vi "DIO - Set Digital Output.vi"(8 "error in":errorcluster, 10 "Channel Number":i32, 11 "TCP Network Connection in":refnum<k5>) -> (0 "error out":errorcluster, 3 "TCP Network Connection out":refnum<k5>)   [LabVIEW 2020]
doc: "Set the state of a digital output. Before setting the state, the channel direction must be set to output."
panel:
  in  "State":bool
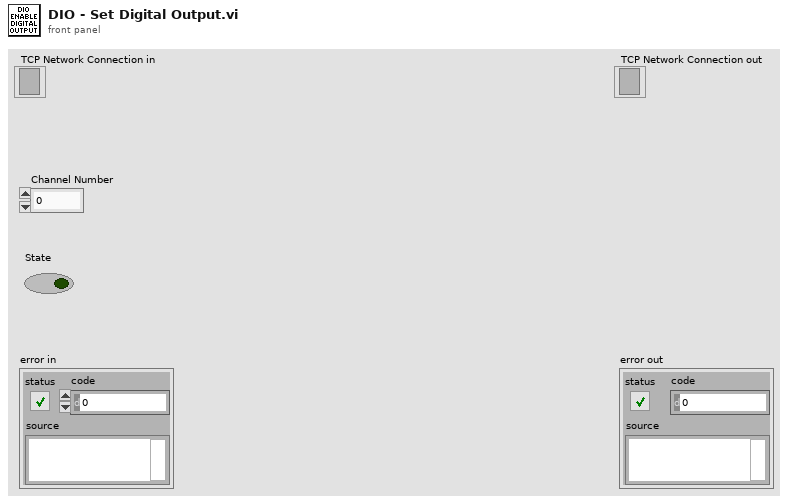
[diagram p1: front panel]
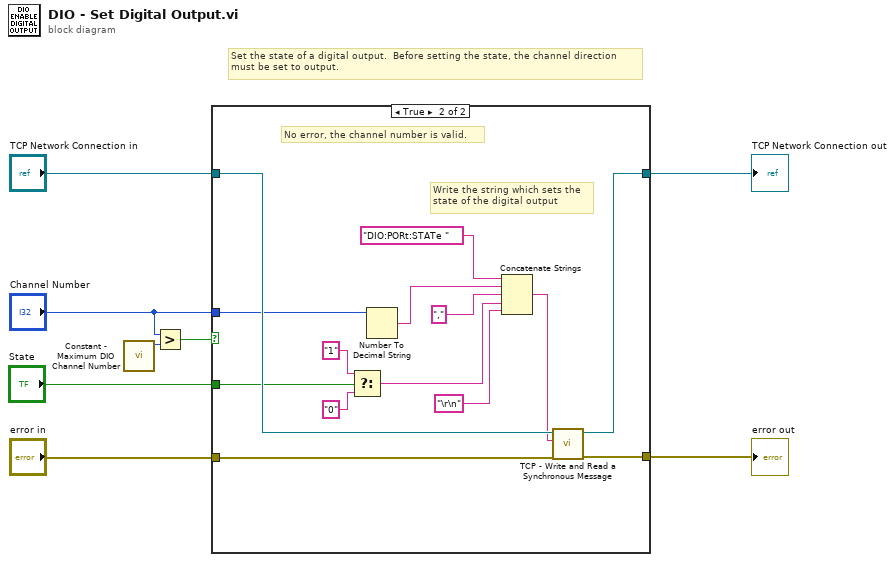
[diagram p0: block diagram]
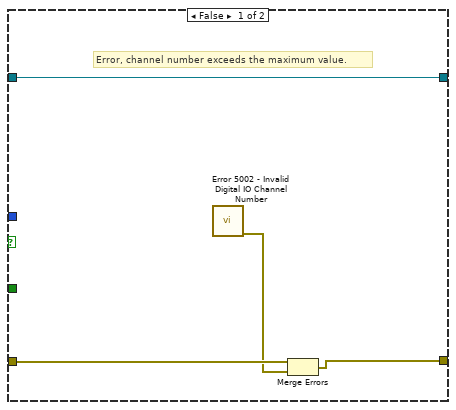
[diagram p2: hidden frame]
diagram:
  # "Set the state of a digital output.  Before setting the state, the channel direction\nmust be set to output."
  n1 = call "Constant - Maximum DIO Channel Number.vi"() -> ("Maximum Channel"=w2:i32)  [unwired: 11 in]
  n2 = Greater?(x="Channel Number", y=w2) -> (0:w1:bool)
  n3 = case shown="True" w1 {
    tunnel: "error in" -> [w12 w26]
    tunnel: "TCP Network Connection in" -> [w9 w25]
    tunnel: [w11 w24] -> w6
    tunnel: [w9 w19] -> w5
    tunnel: "State" -> [_ w18]
    tunnel: "Channel Number" -> [_ w13]
    frame False {
      # "Error, channel number exceeds the maximum value."
      n4 = call "Error 5002 - Invalid Digital IO Channel Number.vi"() -> ("error out"=w10:errorcluster)  [unwired: 11 in]
      n5 = Merge Errors(w12, w10) -> (w11:errorcluster)
    }
    frame True {
      # "Write the string which sets the\nstate of the digital output"
      # "No error, the channel number is valid."
      n6 = Select(t="1", s=w18, f="0") -> (s? t:f=w15:string)
      n7 = Number To Decimal String(number=w13) -> (decimal integer string=w21:string)  [unwired: 1 in]
      n8 = Concatenate Strings("DIO:PORt:STATe " ("Message to Send"), w21, "," ("string"), w15, "\r\n" ("string")) -> (w22:string)
      n9 = call "TCP - Write and Read a Synchronous Message.vi"("error in"=w26, "Message to Send"=w22, "TCP Network Connection in"=w25) -> ("error out"=w24:errorcluster, "TCP Network Connection out"=w19:refnum<k5>)  [unwired: 6 in, 1 out]
    }
  }
  "TCP Network Connection out" <- w5
  "error out" <- w6
